vi "Send Data.vi"(8 "error in (no error)":errorcluster, 10 "Data":u32[](array[numeric]), 11 "FIFO class in":refnum<class "FIFO class.lvclass">) -> (0 "error out":errorcluster, 3 "FIFO class out":refnum<class "FIFO class.lvclass">)   [LabVIEW 2021, in "RT Classes.lvlib" / "FIFO class.lvclass"]
uses:
  FIFO class.lvclass
  FIFO class.lvclass/FIFO class.ctl
  <vilib>/Utility/error.llb/Error Cluster From Error Code.vi
  <vilib>/rvi/errors/niLvFpgaAdjustHostInterfaceError.vi
  <vilib>/rvi/interface/nirviMethod/nirviMethod.xnode
  <vilib>/FPGAPlugInAG/Dynamic/niLvFpga_WriteFifo_Dynamic.vi
  <vilib>/rvi/errors/niLvFpgaMergeErrorWithErrorCode.vi
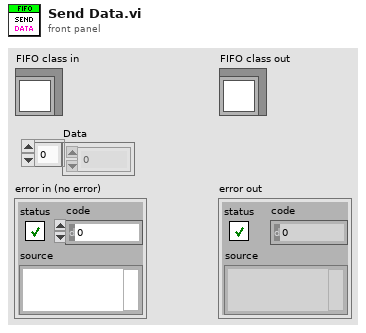
[diagram p1: front panel]
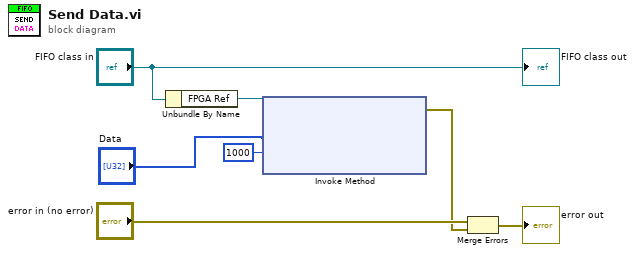
[diagram p0: block diagram]
diagram:
  n1 = Unbundle By Name("FIFO class in") -> ("FPGA Ref"=w5:refnum<k20>)
  n2 = xnode "Invoke Method"("FPGA VI Reference In"=w5, "Data"="Data", "Timeout (ms)"=1000) -> ("error out"=w2:errorcluster)  [unwired: 1 in, 2 out]
  n3 = Merge Errors("error in (no error)", w2) -> (→"error out":errorcluster)
  "FIFO class out" <- "FIFO class in"
